vi "Close.vi"(8 "error in (no error)":errorcluster, 11 "StatD Interface in":refnum<class "StatD Interface.lvclass">) -> (0 "error out":errorcluster)   [LabVIEW 2011, in "StatD Interface.lvclass"]
uses:
  StatD Interface.lvclass
  StatD Interface.lvclass/StatD Interface.ctl
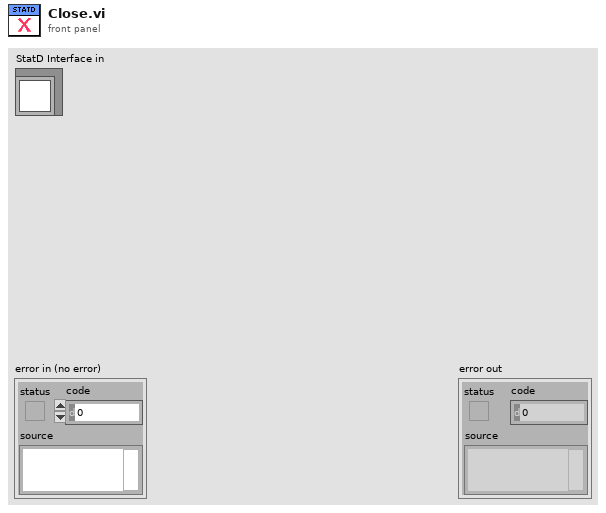
[diagram p1: front panel]
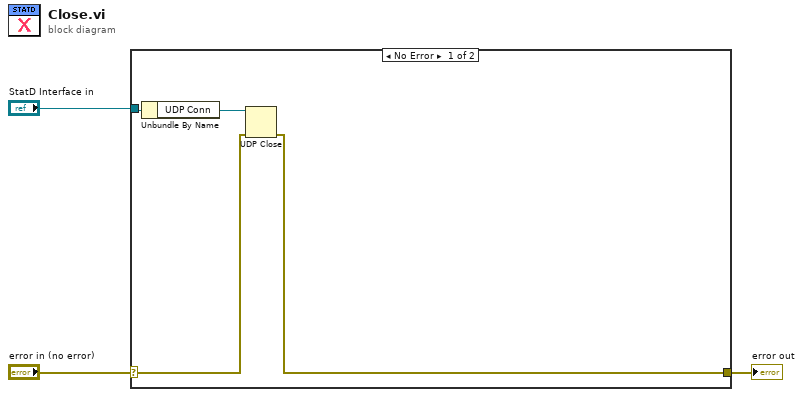
[diagram p0: block diagram]
diagram:
  n1 = case shown="No Error" "error in (no error)" {
    selector: "error in (no error)" -> [w5 w8]
    tunnel: [w4 w8] -> w2
    tunnel: "StatD Interface in" -> [w7 _]
    frame No Error {
      n2 = Unbundle By Name(w7) -> ("UDP Conn"=w6:refnum<k16>)
      n3 = UDP Close(connection ID=w6, 8:w5) -> (error out=w4:errorcluster)  [unwired: 1 out]
    }
    frame Error {
    }
  }
  "error out" <- w2
